vi "SetResolution.vi"(8 "error in (no error)":errorcluster, 10 "Resolution":T1, 11 "CameraTestingProxyAPI in":refnum<class "CameraTestingProxyAPI.lvclass">) -> (0 "error out":errorcluster, 3 "CameraTestingProxyAPI out":refnum<class "CameraTestingProxyAPI.lvclass">)   [LabVIEW 2020, in "CameraTestingProxy.lvlib" / "CameraTestingProxyAPI.lvclass"]
uses:
  CameraTestingProxyAPI.lvclass
  ICameraTestingProxy/TypeDef/Resolution.ctl
  CameraTestingProxyAPI.lvclass/CameraTestingProxyAPI.ctl
  78cdd879-c336-48b0-9ec9-8e8fd70fc643.vi
  ICameraTestingProxy/TypeDef/ICameraTestingProxy_typedef.lvlib
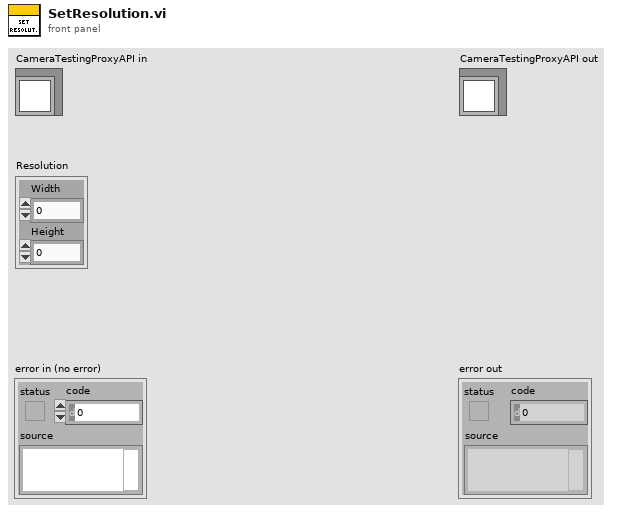
[diagram p1: front panel]
types:
  T1 = typedef "ICameraTestingProxy_typedef.lvlib/Resolution.ctl" = cluster{"Width":i16, "Height":i16}
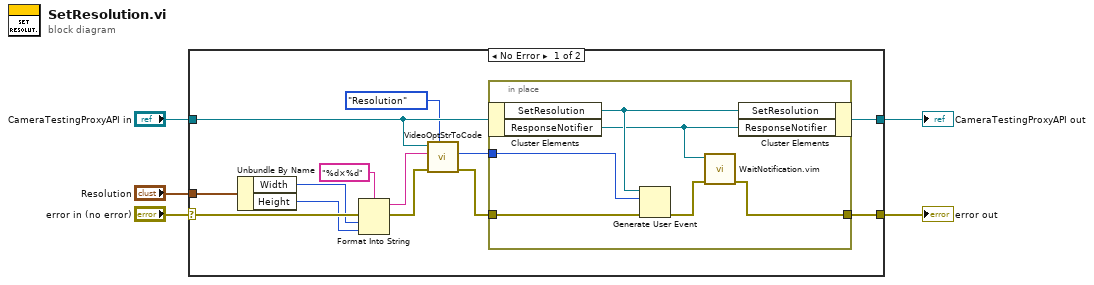
[diagram p0: block diagram]
diagram:
  n1 = case shown="No Error" "error in (no error)" {
    selector: "error in (no error)" -> [w13 w26]
    tunnel: "CameraTestingProxyAPI in" -> [w16 w25]
    tunnel: [w18 w26] -> w3
    tunnel: [w17 w25] -> w2
    tunnel: "Resolution" -> [w10 _]
    frame No Error {
      n2 = Unbundle By Name(w10) -> ("Width"=w7:i16, "Height"=w6:i16)
      n3 = Format Into String(format string="%d×%d", error in=w13, w7, w6) -> (resulting string=w14:string, error out=w12:errorcluster)  [unwired: 1 in]
      n4 = call "VideoOptStrToCode.vi"("VideoOption"=enum16{"FrameRate", "ImageType", "Resolution"}."Resolution", "error in (no error)"=w12, "DescriptionString"=w14, "CameraTestingProxyAPI in"=w16) -> ("error out"=w11:errorcluster, "Code"=w15:u8)  [unwired: 5 in, 1 out]
      n5 = in-place {
        in-place-border: w11 -> [w24]
        in-place-border: [w20] -> w18
        in-place-border: w15 -> [w22]
        n6 = in-place-cluster #1(w16) -> ("SetResolution"=w23:refnum<user-event>, "ResponseNotifier"=w19:refnum<notifier>)
        n7 = Generate User Event(user event=w23, event data cluster=w22, error in=w24) -> (error out=w21:errorcluster)  [unwired: 1 in, 1 out]
        n8 = call "WaitNotification.vim"("error in (no error)"=w21, "ResponseNotifier"=w19) -> ("error out"=w20:errorcluster)  [unwired: 8 in, 1 out]
        n9 = in-place-cluster #1("SetResolution"=w23, "ResponseNotifier"=w19) -> (w17:refnum<class "CameraTestingProxyAPI.lvclass">)
      }
    }
    frame Error {
    }
  }
  "error out" <- w3
  "CameraTestingProxyAPI out" <- w2
